vi "_DP2TDMProperties.vi"(8 "error in (no error)":errorcluster, 10 "DataPlugin Object in":refnum<k20>, 11 "TDM Object in":refnum<k20>) -> (0 "error out":errorcluster, 2 "DataPlugin object out":refnum<k20>, 3 "TDM Object out":refnum<k20>)   [LabVIEW 2017]
uses:
  <vilib>/Platform/storage/Storage.llb/Get Property (I16).vi
  <vilib>/Platform/storage/Storage.llb/Set Property (I16).vi
  <vilib>/Platform/storage/Storage.llb/Get Property (I32).vi
  <vilib>/Platform/storage/Storage.llb/Set Property (I32).vi
  <vilib>/Platform/storage/Storage.llb/Get Property (DBL).vi
  <vilib>/Platform/storage/Storage.llb/Set Property (DBL).vi
  <vilib>/Platform/storage/Storage.llb/Get Property (U8).vi
  <vilib>/Platform/storage/Storage.llb/Set Property (U8).vi
  <vilib>/Platform/storage/Storage.llb/Get Property (SGL).vi
  <vilib>/Platform/storage/Storage.llb/Set Property (SGL).vi
  <vilib>/Platform/storage/Storage.llb/Get Property (String).vi
  <vilib>/Platform/storage/Storage.llb/Set Property (String).vi
  <vilib>/Platform/storage/Storage.llb/Get Property (Time Stamp).vi
  <vilib>/Platform/storage/Storage.llb/Set Property (Time Stamp).vi
  <vilib>/Platform/storage/Storage.llb/Get Property (Enum).vi
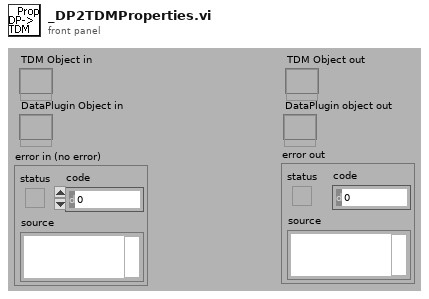
[diagram p1: front panel]
types:
  T1 = typedef "usiProperty.ctl" = cluster{"object type":T2, "property name":string, "data type":T3}
  T2 = typedef "usiObjectType.ctl" = enum16{"File", "Channel Group", "Channel", "Unknown"}
  T3 = typedef "usiDataType.ctl" = enum16{"eNoTypeUsi", "eInt8Usi", "eInt16Usi", "eInt32Usi", "eInt64Usi", "eUInt8Usi", "eUInt16Usi", "eUInt32Usi", "eUInt64Usi", "eFloat32Usi", "eFloat64Usi", "- 0", "- 1", "- 2", "- 3", "- 4", "- 5", "- 6", "- 7", "- 8", "- 9", "eString8Usi", "eString16Usi", "eStringUsi", "eEnumUsi", "- 10", "- 11", "- 12", "- 13", "- 14", "eTimeUsi", "- 15", "- 16", "- 17", "- 18", "- 19", "- 20", "- 21", "- 22", "- 23", "eInstanceUsi", "eStoreUsi"}
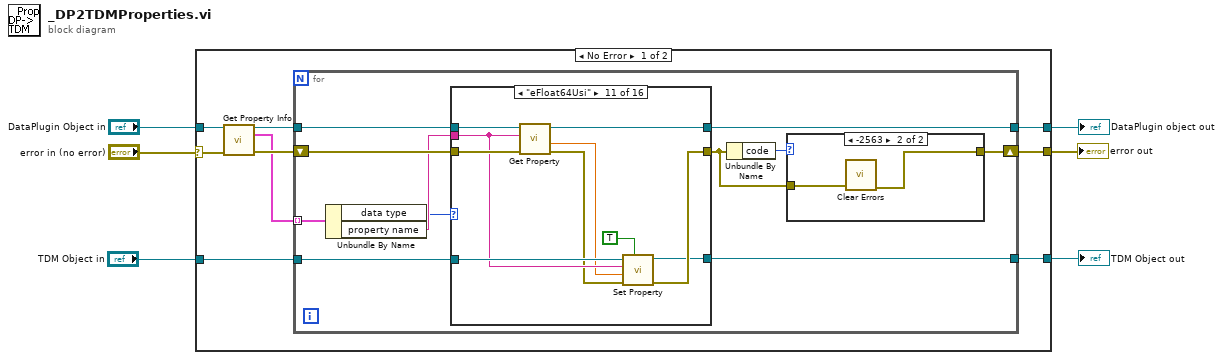
[diagram p0: block diagram]
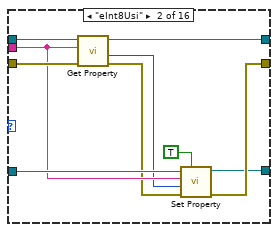
[diagram p4: hidden frame]
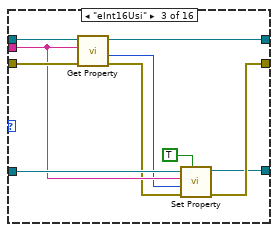
[diagram p5: hidden frame]
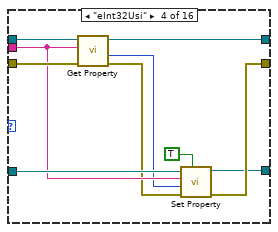
[diagram p6: hidden frame]
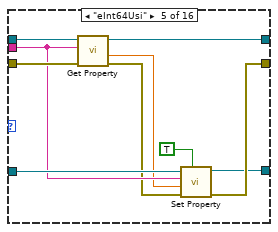
[diagram p7: hidden frame]
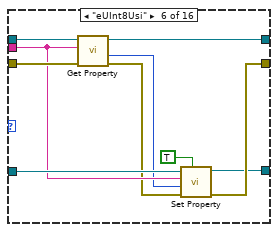
[diagram p8: hidden frame]
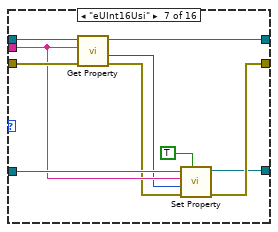
[diagram p9: hidden frame]
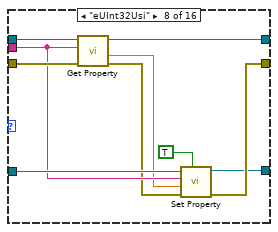
[diagram p10: hidden frame]
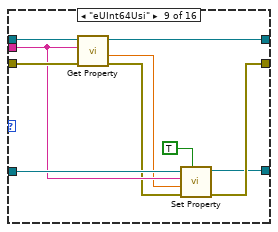
[diagram p11: hidden frame]
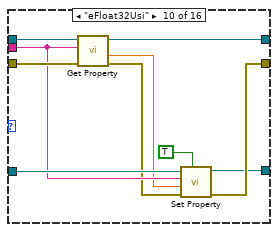
[diagram p12: hidden frame]
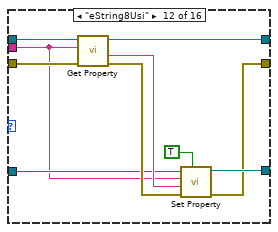
[diagram p13: hidden frame]
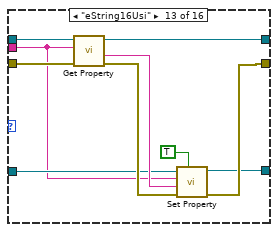
[diagram p14: hidden frame]
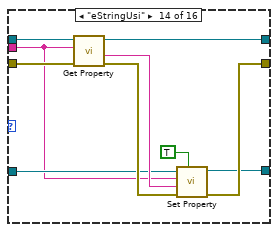
[diagram p15: hidden frame]
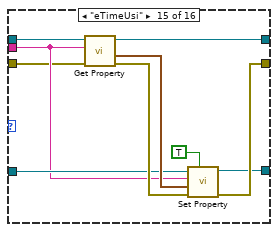
[diagram p16: hidden frame]
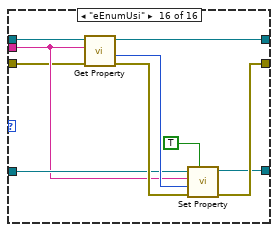
[diagram p17: hidden frame]
diagram:
  n1 = case shown="No Error" "error in (no error)" {
    selector: "error in (no error)" -> [w14 w185]
    tunnel: "DataPlugin Object in" -> [w15 w184]
    tunnel: [w8 w184] -> w5
    tunnel: [w12 w185] -> w4
    tunnel: "TDM Object in" -> [w9 w183]
    tunnel: [w7 w183] -> w1
    frame No Error {
      n2 = call <vilib>:"Get Property Info.vi"("storage refnum"=w15, "error in (no error)"=w14) -> ("storage refnum out"=w10:refnum<k20>, "properties"=w11:T1[], "error out"=w13:errorcluster)  [unwired: 11 in]
      n3 = for {
        shift-right: [w16] -> w12
        shift-left: w13 -> [w26]
        tunnel: w11 -> [w25] mode=indexing
        tunnel: w10 -> [w21]
        tunnel: w9 -> [w22]
        tunnel: [w20] -> w8
        tunnel: [w19] -> w7
        n4 = Unbundle By Name(w25) -> ("data type"=w23:T3, "property name"=w24:string)
        n5 = case shown="\"eFloat64Usi\"" w23 {
          tunnel: w26 -> [w31 w42 w52 w62 w72 w82 w92 w102 w112 w122 w132 w138 w144 w154 w164 w175]
          tunnel: w24 -> [_ w39 w49 w59 w69 w79 w89 w99 w109 w119 w129 w136 w143 w153 w165 w176]
          tunnel: w22 -> [w30 w40 w50 w60 w70 w80 w90 w100 w110 w120 w130 w137 w146 w156 w166 w177]
          tunnel: w21 -> [w32 w41 w51 w61 w71 w81 w91 w101 w111 w121 w131 w139 w145 w155 w163 w174]
          tunnel: [w31 w36 w46 w56 w66 w76 w86 w96 w106 w116 w126 w133 w148 w158 w169 w180] -> w17
          tunnel: [w32 w35 w45 w55 w65 w75 w85 w95 w105 w115 w125 w140 w149 w159 w168 w179] -> w20
          tunnel: [w30 w34 w44 w54 w64 w74 w84 w94 w104 w114 w124 w135 w147 w157 w167 w178] -> w19
          frame "eNoTypeUsi", Default {
          }
          frame "eInt8Usi" {
            n6 = call-poly <vilib>:"Get Property.vi"("error in (no error)"=w42, "Property name"=w39, "storage refnum"=w41) -> ("error out"=w37:errorcluster, "Value"=w38:i16, "storage refnum out"=w35:refnum<k20>)  [unwired: 6 in]
            n7 = call-poly <vilib>:"Set Property.vi"("Create if not found (no:F)"=TRUE, "error in (no error)"=w37, "Value"=w38, "Property name"=w39, "storage refnum"=w40) -> ("error out"=w36:errorcluster, "storage refnum out"=w34:refnum<k20>)  [unwired: 5 in]
          }
          frame "eInt16Usi" {
            n8 = call-poly <vilib>:"Get Property.vi"("error in (no error)"=w52, "Property name"=w49, "storage refnum"=w51) -> ("error out"=w47:errorcluster, "Value"=w48:i16, "storage refnum out"=w45:refnum<k20>)  [unwired: 6 in]
            n9 = call-poly <vilib>:"Set Property.vi"("Create if not found (no:F)"=TRUE, "error in (no error)"=w47, "Value"=w48, "Property name"=w49, "storage refnum"=w50) -> ("error out"=w46:errorcluster, "storage refnum out"=w44:refnum<k20>)  [unwired: 5 in]
          }
          frame "eInt32Usi" {
            n10 = call-poly <vilib>:"Get Property.vi"("error in (no error)"=w62, "Property name"=w59, "storage refnum"=w61) -> ("error out"=w57:errorcluster, "Value"=w58:i32, "storage refnum out"=w55:refnum<k20>)  [unwired: 6 in]
            n11 = call-poly <vilib>:"Set Property.vi"("Create if not found (no:F)"=TRUE, "error in (no error)"=w57, "Value"=w58, "Property name"=w59, "storage refnum"=w60) -> ("error out"=w56:errorcluster, "storage refnum out"=w54:refnum<k20>)  [unwired: 5 in]
          }
          frame "eInt64Usi" {
            n12 = call-poly <vilib>:"Get Property.vi"("error in (no error)"=w72, "Property name"=w69, "storage refnum"=w71) -> ("error out"=w67:errorcluster, "Value"=w68:dbl, "storage refnum out"=w65:refnum<k20>)  [unwired: 6 in]
            n13 = call-poly <vilib>:"Set Property.vi"("Create if not found (no:F)"=TRUE, "error in (no error)"=w67, "Value"=w68, "Property name"=w69, "storage refnum"=w70) -> ("error out"=w66:errorcluster, "storage refnum out"=w64:refnum<k20>)  [unwired: 5 in]
          }
          frame "eUInt8Usi" {
            n14 = call-poly <vilib>:"Get Property.vi"("error in (no error)"=w82, "Property name"=w79, "storage refnum"=w81) -> ("error out"=w77:errorcluster, "Value"=w78:u8, "storage refnum out"=w75:refnum<k20>)  [unwired: 6 in]
            n15 = call-poly <vilib>:"Set Property.vi"("Create if not found (no:F)"=TRUE, "error in (no error)"=w77, "Value"=w78, "Property name"=w79, "storage refnum"=w80) -> ("error out"=w76:errorcluster, "storage refnum out"=w74:refnum<k20>)  [unwired: 5 in]
          }
          frame "eUInt16Usi" {
            n16 = call-poly <vilib>:"Get Property.vi"("error in (no error)"=w92, "Property name"=w89, "storage refnum"=w91) -> ("error out"=w87:errorcluster, "Value"=w88:i32, "storage refnum out"=w85:refnum<k20>)  [unwired: 6 in]
            n17 = call-poly <vilib>:"Set Property.vi"("Create if not found (no:F)"=TRUE, "error in (no error)"=w87, "Value"=w88, "Property name"=w89, "storage refnum"=w90) -> ("error out"=w86:errorcluster, "storage refnum out"=w84:refnum<k20>)  [unwired: 5 in]
          }
          frame "eUInt32Usi" {
            n18 = call-poly <vilib>:"Get Property.vi"("error in (no error)"=w102, "Property name"=w99, "storage refnum"=w101) -> ("error out"=w97:errorcluster, "Value"=w98:dbl, "storage refnum out"=w95:refnum<k20>)  [unwired: 6 in]
            n19 = call-poly <vilib>:"Set Property.vi"("Create if not found (no:F)"=TRUE, "error in (no error)"=w97, "Value"=w98, "Property name"=w99, "storage refnum"=w100) -> ("error out"=w96:errorcluster, "storage refnum out"=w94:refnum<k20>)  [unwired: 5 in]
          }
          frame "eUInt64Usi" {
            n20 = call-poly <vilib>:"Get Property.vi"("error in (no error)"=w112, "Property name"=w109, "storage refnum"=w111) -> ("error out"=w107:errorcluster, "Value"=w108:dbl, "storage refnum out"=w105:refnum<k20>)  [unwired: 6 in]
            n21 = call-poly <vilib>:"Set Property.vi"("Create if not found (no:F)"=TRUE, "error in (no error)"=w107, "Value"=w108, "Property name"=w109, "storage refnum"=w110) -> ("error out"=w106:errorcluster, "storage refnum out"=w104:refnum<k20>)  [unwired: 5 in]
          }
          frame "eFloat32Usi" {
            n22 = call-poly <vilib>:"Get Property.vi"("error in (no error)"=w122, "Property name"=w119, "storage refnum"=w121) -> ("error out"=w117:errorcluster, "Value"=w118:sgl, "storage refnum out"=w115:refnum<k20>)  [unwired: 6 in]
            n23 = call-poly <vilib>:"Set Property.vi"("Create if not found (no:F)"=TRUE, "error in (no error)"=w117, "Value"=w118, "Property name"=w119, "storage refnum"=w120) -> ("error out"=w116:errorcluster, "storage refnum out"=w114:refnum<k20>)  [unwired: 5 in]
          }
          frame "eFloat64Usi" {
            n24 = call-poly <vilib>:"Get Property.vi"("error in (no error)"=w132, "Property name"=w129, "storage refnum"=w131) -> ("error out"=w127:errorcluster, "Value"=w128:dbl, "storage refnum out"=w125:refnum<k20>)  [unwired: 6 in]
            n25 = call-poly <vilib>:"Set Property.vi"("Create if not found (no:F)"=TRUE, "error in (no error)"=w127, "Value"=w128, "Property name"=w129, "storage refnum"=w130) -> ("error out"=w126:errorcluster, "storage refnum out"=w124:refnum<k20>)  [unwired: 5 in]
          }
          frame "eString8Usi" {
            n26 = call-poly <vilib>:"Get Property.vi"("error in (no error)"=w138, "Property name"=w136, "storage refnum"=w139) -> ("error out"=w141:errorcluster, "Value"=w142:string, "storage refnum out"=w140:refnum<k20>)  [unwired: 6 in]
            n27 = call-poly <vilib>:"Set Property.vi"("Create if not found (no:F)"=TRUE, "error in (no error)"=w141, "Value"=w142, "Property name"=w136, "storage refnum"=w137) -> ("error out"=w133:errorcluster, "storage refnum out"=w135:refnum<k20>)  [unwired: 5 in]
          }
          frame "eString16Usi" {
            n28 = call-poly <vilib>:"Get Property.vi"("error in (no error)"=w144, "Property name"=w143, "storage refnum"=w145) -> ("error out"=w151:errorcluster, "Value"=w152:string, "storage refnum out"=w149:refnum<k20>)  [unwired: 6 in]
            n29 = call-poly <vilib>:"Set Property.vi"("Create if not found (no:F)"=TRUE, "error in (no error)"=w151, "Value"=w152, "Property name"=w143, "storage refnum"=w146) -> ("error out"=w148:errorcluster, "storage refnum out"=w147:refnum<k20>)  [unwired: 5 in]
          }
          frame "eStringUsi" {
            n30 = call-poly <vilib>:"Get Property.vi"("error in (no error)"=w154, "Property name"=w153, "storage refnum"=w155) -> ("error out"=w161:errorcluster, "Value"=w162:string, "storage refnum out"=w159:refnum<k20>)  [unwired: 6 in]
            n31 = call-poly <vilib>:"Set Property.vi"("Create if not found (no:F)"=TRUE, "error in (no error)"=w161, "Value"=w162, "Property name"=w153, "storage refnum"=w156) -> ("error out"=w158:errorcluster, "storage refnum out"=w157:refnum<k20>)  [unwired: 5 in]
          }
          frame "eTimeUsi" {
            n32 = call-poly <vilib>:"Get Property.vi"("error in (no error)"=w164, "Property name"=w165, "storage refnum"=w163) -> ("error out"=w171:errorcluster, "Value"=w172:timestamp, "storage refnum out"=w168:refnum<k20>)  [unwired: 6 in]
            n33 = call-poly <vilib>:"Set Property.vi"("Create if not found (no:F)"=TRUE, "error in (no error)"=w171, "Value"=w172, "Property name"=w165, "storage refnum"=w166) -> ("error out"=w169:errorcluster, "storage refnum out"=w167:refnum<k20>)  [unwired: 5 in]
          }
          frame "eEnumUsi" {
            n34 = call-poly <vilib>:"Get Property.vi"("error in (no error)"=w175, "Property name"=w176, "storage refnum"=w174) -> ("error out"=w181:errorcluster, "Value"=w182:u16, "storage refnum out"=w179:refnum<k20>)  [unwired: 5 in, 1 out]
            n35 = call-poly <vilib>:"Set Property.vi"("Create if not found (no:F)"=TRUE, "error in (no error)"=w181, "Value"=w182, "Property name"=w176, "storage refnum"=w177) -> ("error out"=w180:errorcluster, "storage refnum out"=w178:refnum<k20>)  [unwired: 5 in]
          }
        }
        n36 = Unbundle By Name(w17) -> ("code"=w18:i32)
        n37 = case shown="-2563" w18 {
          tunnel: w17 -> [w27 w29]
          tunnel: [w27 w28] -> w16
          frame Default {
          }
          frame -2563 {
            n38 = call <vilib>:"Clear Errors.vi"("error in (no error)"=w29) -> ("error out"=w28:errorcluster)  [unwired: 5 in, 1 out]
          }
        }
      }
    }
    frame Error {
    }
  }
  "DataPlugin object out" <- w5
  "error out" <- w4
  "TDM Object out" <- w1
